vi "DPOAE-CPMR-3.vi"() -> ()   [LabVIEW 2014]
uses:
  <vilib>/measure/NI_MABase.lvlib
  <vilib>/DAQmx/configure/trigger.llb/DAQmx Start Trigger (Digital Edge).vi
  <vilib>/DAQmx/configure/timing.llb/DAQmx Timing (Sample Clock).vi
  <vilib>/DAQmx/create/channels.llb/DAQmx Create Channel (AO-Voltage-Basic).vi
  <vilib>/DAQmx/read.llb/DAQmx Read (Analog Wfm 1Chan NSamp).vi
  <resource>/objmgr/daqmx.rc
  <vilib>/DAQmx/write.llb/DAQmx Write (Analog 1D Wfm NChan NSamp).vi
  <vilib>/DAQmx/create/channels.llb/DAQmx Create Channel (AI-Sound Pressure-Microphone).vi
panel:
  out "Test settings str":string[][](array[string])
  out "Expinfo words":string[](array[string])
  in  "Stop!":bool
  out "End of test":bool
  out "Theoretical freq DPOAE (kHz)":dbl
  out "Frequency Spectrum":cluster{"x0":dbl, "dx":dbl, "magnitude":dbl[]}(graph) caption="spectrum"
  in  "Frequency 2 (kHz)":dbl(ring)=2000.0 items=["0"=0.0, "2"=2000.0, "3"=3000.0, "4"=4000.0, "5"=5000.0, "6"=6000.0, "7"=7000.0, "8"=8000.0, "9"=9000.0, "10"=10000.0, "11"=11000.0, "12"=12000.0, "16"=16000.0]
  out "Stimulus 2 Graph":waveform(dbl)(graph)
  in  "Output Channels (Select two):":tag="PXI1Slot6/ao0:1"
  in  "Amplitude 2":u16(ring)=50 items=["50"=50, "55"=55, "60"=60, "65"=65, "70"=70]
  in  "Add Button 2":bool
  out "Amplitude 1":u16
  out "Frequency 1 (kHz)":dbl=13333.333333333334 format="%#.2f"
  out "Date_Time":string
  out "Main file name":string[](array[string])
  out "Fs":string
  out "File path str":string
  in  "Subject ID":string
  out "Expinfo name":string[](array[string])
  out "File name":string[](array[string])
  in  "File path":path
  in  "User name":string
  in  "Start!":bool
  out "Acquisition Graph":waveform(dbl)(graph)
  in  "Input Channel":tag="PXI1Slot6/ai0"
  out "Fs (#S/s)":dbl
  out "Stimulus 1 Graph":waveform(dbl)(graph)
  out "Current test":i32(knob) scale=0.0..10.0
  in  "Sampling info":cluster{"Fs (#S/s)":dbl, "#S":dbl}={"Fs (#S/s)"=96000.0, "#S"=200000.0}
  out "Protocol list":string[](array[string])
  out "Protocol array settings":dbl[][](array[numeric])
  out "iteration":i32
  in  "How many tests?":i32(slide) scale=0.0..10.0
  out "Protocol words":string[](array[string])
  out "Test settings":dbl[](array[numeric])
  # "Protocol list:"
  # "User, Subject and File settings:"
  # "1"
  # "(without spaces)"
  # "(without spaces)"
  # "(without spaces)"
  # "2"
  # "Choose channels:"
  # "3"
  # "Select sample rate:"
  # "Protocol settings:"
  # "4"
  # "5"
  # "Add a final F2 = 0 kHz stimulus to record noise level."
  # "6"
  # "7"
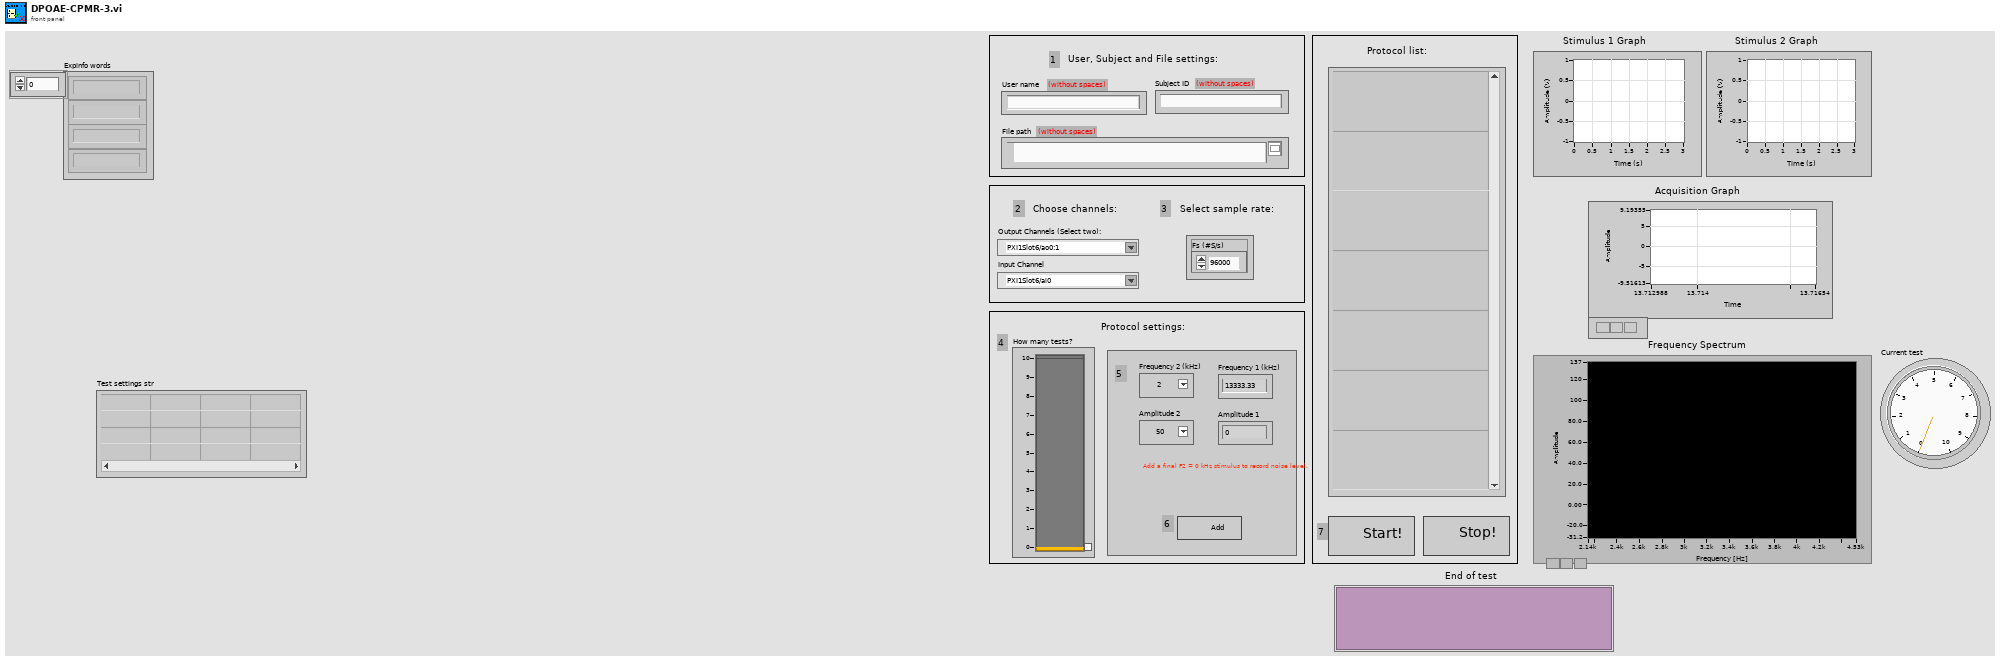
[diagram p1: front panel]
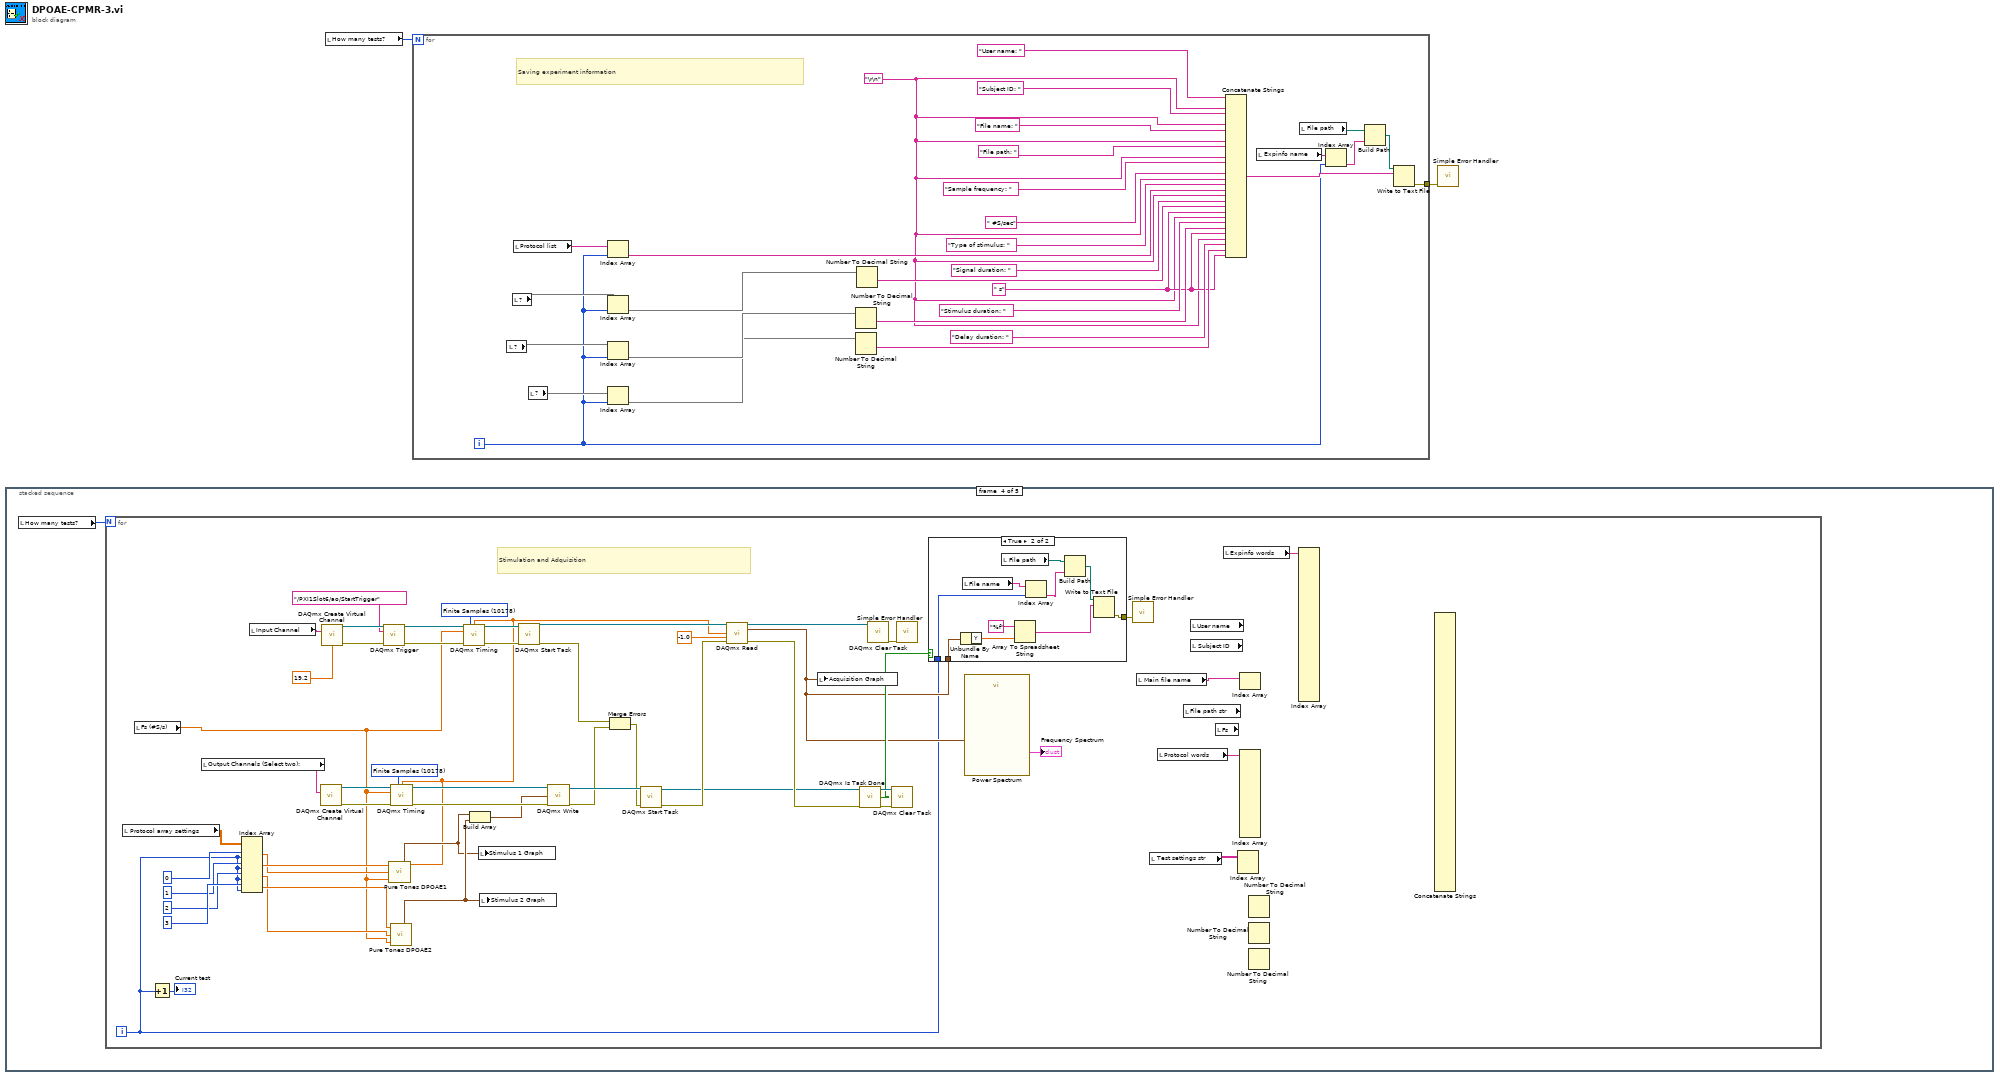
[diagram p0: block diagram]
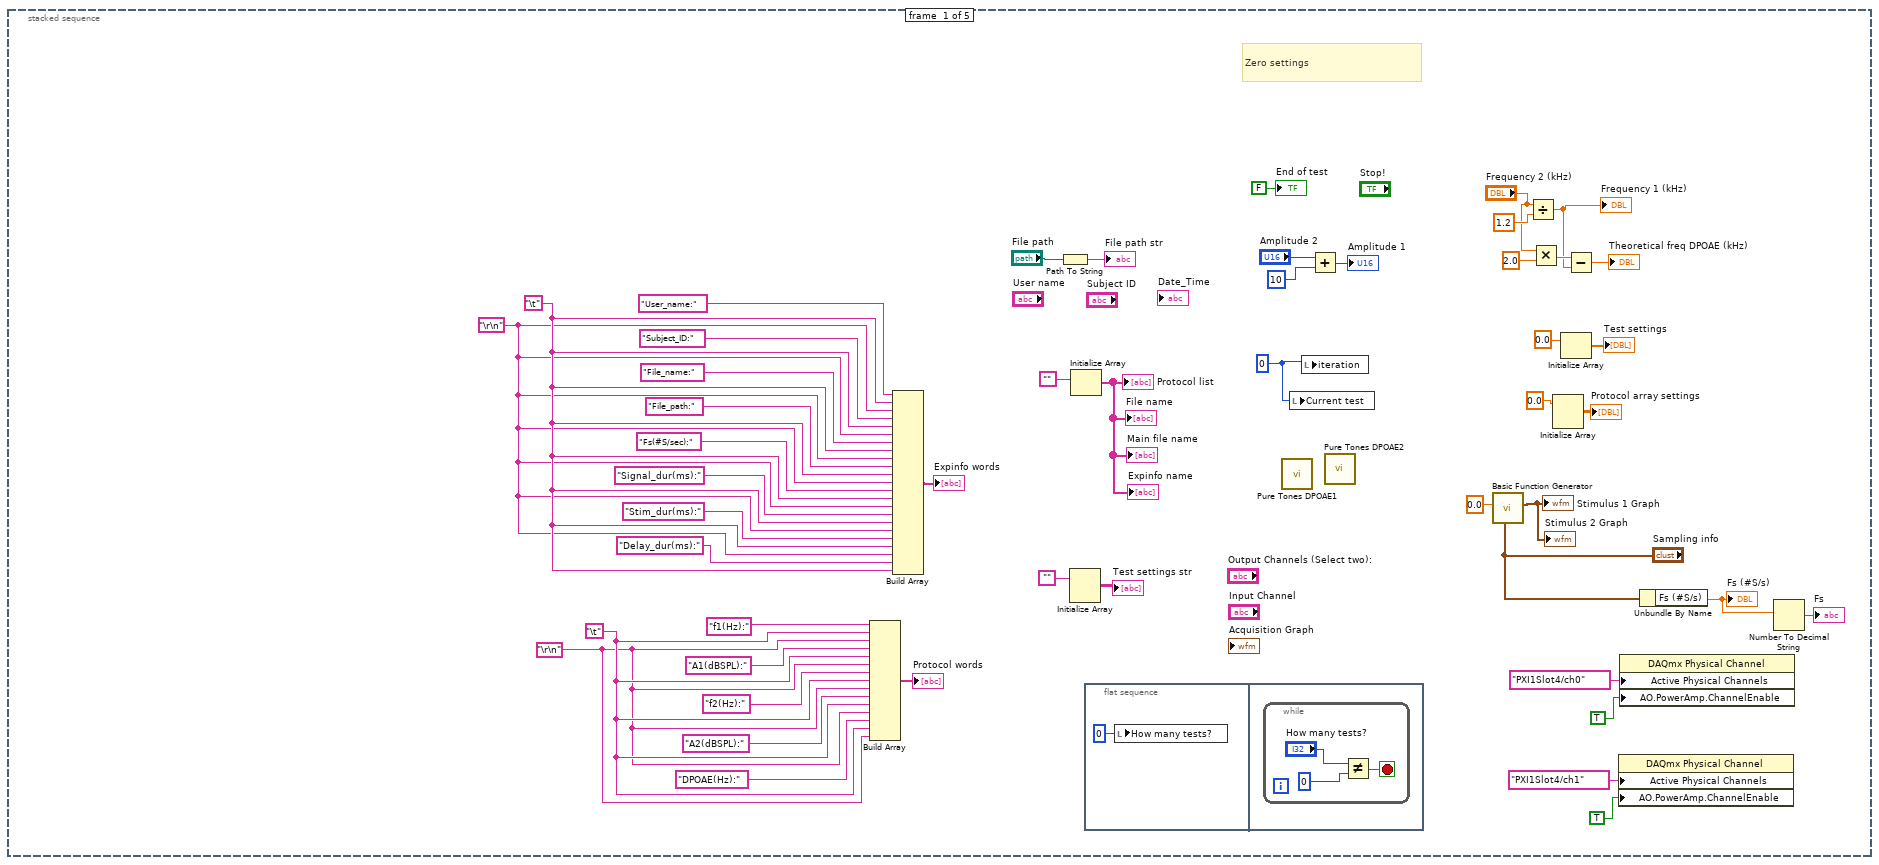
[diagram p2: hidden frame]
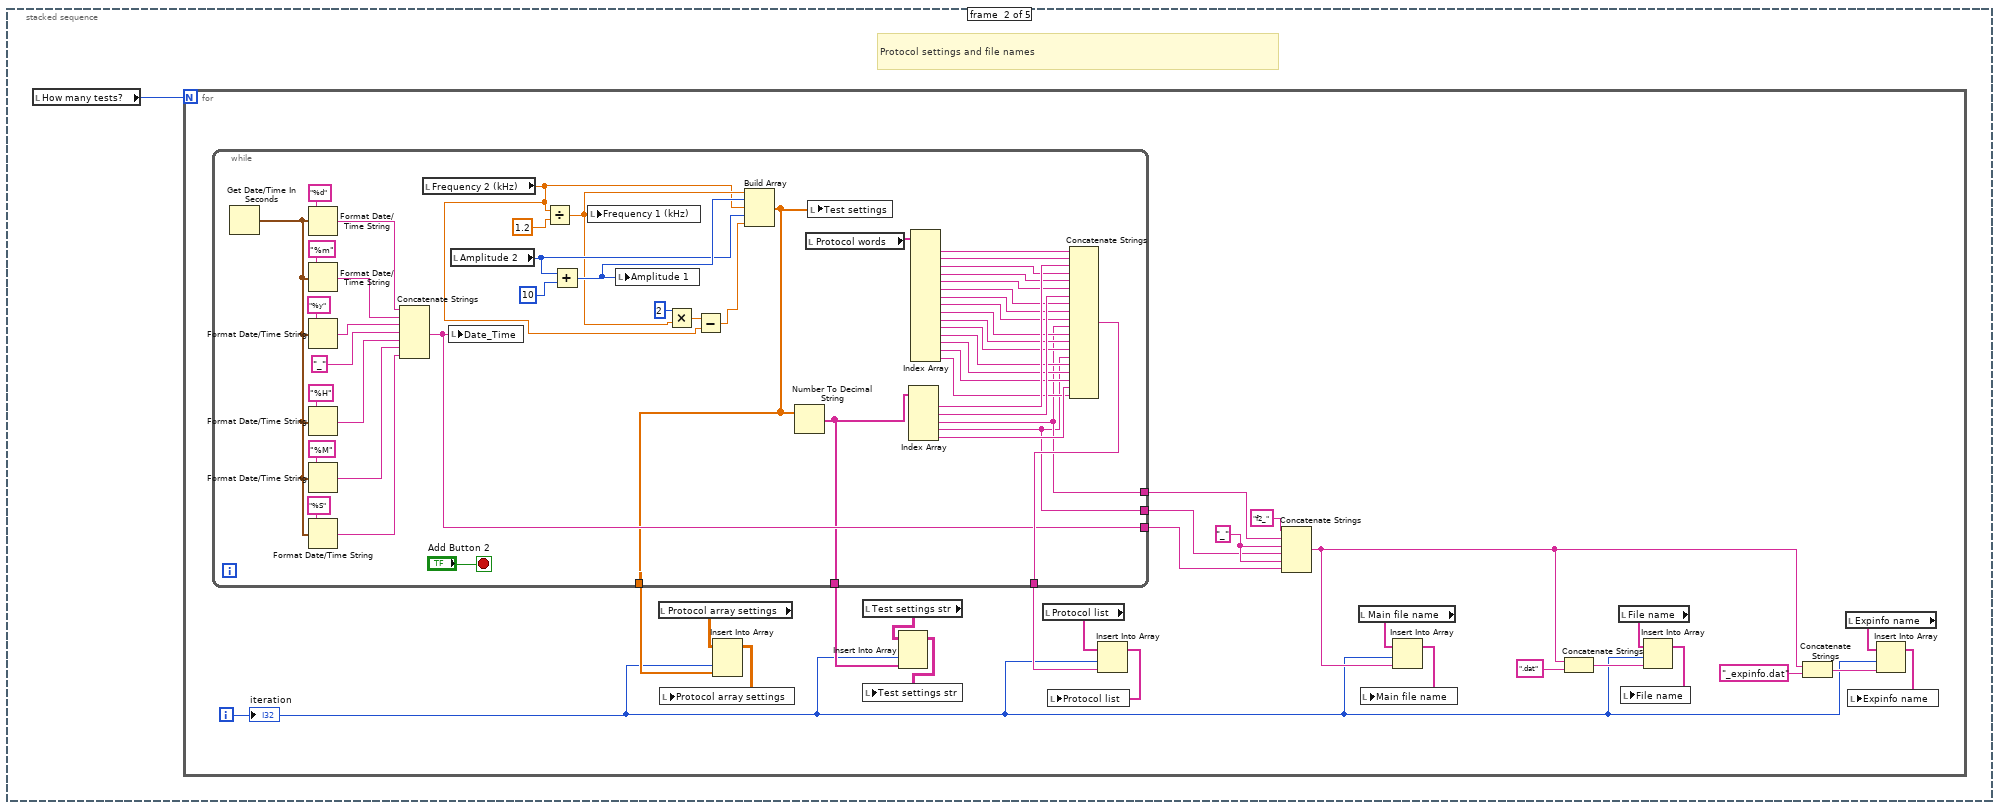
[diagram p3: hidden frame]
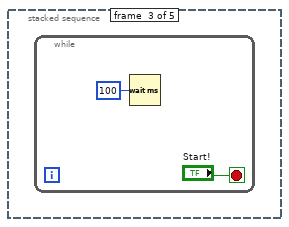
[diagram p4: hidden frame]
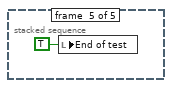
[diagram p6: hidden frame]
diagram:
  n1 = stacked-sequence {
    frame #0 {
      w7 = "\t"
      w6 = "\r\n"
      w11 = "\t"
      w10 = "\r\n"
      w45 = 0 ("iteration")
      # "Zero settings"
      n2 = Build Array("f1(Hz):" ("string"), w7, w6, "A1(dBSPL):", w7, w6, "f2(Hz):" ("string"), w7, w6, "A2(dBSPL):" ("string"), w7, w6, "DPOAE(Hz):" ("string"), w7, w6) -> (→"Protocol words":string[])
      n3 = Build Array("User_name:", w11, w10, "Subject_ID:", w11, w10, "File_name:", w11, w10, "File_path:", w11, w10, "Fs(#S/sec):", w11, w10, "Signal_dur(ms):", w11, w10, "Stim_dur(ms):", w11, w10, "Delay_dur(ms):", w11) -> (→"Expinfo words":string[])
      n4 = Path To String(path="File path") -> (string=→"File path str":string)
      n5 = Initialize Array("") -> (→"Test settings str":string[][])  [unwired: 2 in]
      n6 = Initialize Array("") -> (→"Protocol list" →"File name" →"Expinfo name" →"Main file name":string[])  [unwired: 1 in]
      n7 = flat-sequence {
        frame #0 {
          n8 = local write "How many tests?"(0 ("How many tests?")) -> ()
        }
        frame #1 {
          n9 = while {
            stop <- w54 stop-if-true
            n10 = Not Equal?(x="How many tests?", y=0) -> (x != y?=w54:bool)
          }
        }
      }
      n11 = call <userlib>:"Pure Tones DPOAE1.vi"() -> ()  [unwired: 3 in, 5 out]
      n12 = local write "Current test"(w45) -> ()
      n13 = local write "iteration"(w45) -> ()
      n14 = Add(x="Amplitude 2", y=10) -> (x+y=→"Amplitude 1":i32)
      n15 = call <userlib>:"Pure Tones DPOAE2.vi"() -> ()  [unwired: 3 in, 5 out]
      n16 = call <vilib>:"Basic Function Generator.vi"("sampling info"="Sampling info", "amplitude"=0.0) -> ("signal out"=→"Stimulus 1 Graph" →"Stimulus 2 Graph":waveform(dbl))  [unwired: 7 in, 2 out]
      n17 = Divide(x="Frequency 2 (kHz)", y=1.2) -> (x/y=w26:dbl)
      "Frequency 1 (kHz)" <- w26
      n18 = Multiply(x="Frequency 2 (kHz)", y=2.0) -> (x*y=w27:dbl)
      n19 = Initialize Array(0.0 ("element")) -> (→"Protocol array settings":dbl[][])  [unwired: 2 in]
      n20 = Initialize Array(0.0 ("element")) -> (→"Test settings":dbl[])  [unwired: 1 in]
      n21 = Subtract(x=w27, y=w26) -> (x-y=→"Theoretical freq DPOAE (kHz)":dbl)
      n22 = property class="DAQmx Physical Channel"("Active Physical Channels"=tag "PXI1Slot4/ch1" ("ActivePhysicalChans"), "AO.PowerAmp.ChannelEnable"=TRUE) -> ()  [unwired: 2 in, 2 out]
      n23 = property class="DAQmx Physical Channel"("Active Physical Channels"=tag "PXI1Slot4/ch0" ("ActivePhysicalChans"), "AO.PowerAmp.ChannelEnable"=TRUE) -> ()  [unwired: 2 in, 2 out]
      n24 = Unbundle By Name("Sampling info") -> ("Fs (#S/s)"=w41:dbl)
      "Fs (#S/s)" <- w41
      n25 = Number To Decimal String(number=w41) -> (decimal integer string=→"Fs":string)  [unwired: 1 in]
      "End of test" <- FALSE ("End of test")
    }
    frame #1 {
      # "Protocol settings and file names"
      n26 = local read "How many tests?"() -> (w56:i32)
      n27 = for {
        N: w56 -> [_]
        i -> [w58]
        w72 = "_"
        n28 = while {
          tunnel: [w131] -> w73
          tunnel: [w112] -> w78
          tunnel: [w83] -> w70
          tunnel: [w84] -> w71
          tunnel: [w116] -> w69
          tunnel: [w85] -> w59
          stop <- "Add Button 2" stop-if-true
          n29 = Get Date/Time In Seconds() -> (seconds since 1Jan1904=w123:timestamp)
          n30 = Format Date/Time String(time format string (%c)="%d", seconds (now)=w123) -> (date/time string=w124:string)  [unwired: 1 in]
          n31 = Format Date/Time String(time format string (%c)="%m", seconds (now)=w123) -> (date/time string=w125:string)  [unwired: 1 in]
          n32 = Format Date/Time String(time format string (%c)="%y", seconds (now)=w123) -> (date/time string=w126:string)  [unwired: 1 in]
          n33 = Format Date/Time String(time format string (%c)="%H", seconds (now)=w123) -> (date/time string=w127:string)  [unwired: 1 in]
          n34 = Format Date/Time String(time format string (%c)="%M", seconds (now)=w123) -> (date/time string=w128:string)  [unwired: 1 in]
          n35 = Format Date/Time String(time format string (%c)="%S", seconds (now)=w123) -> (date/time string=w129:string)  [unwired: 1 in]
          n36 = Concatenate Strings(w124, w125, w126, "_", w127, w128, w129) -> (w116:string)
          n37 = local read "Frequency 2 (kHz)"() -> (w106:dbl)
          n38 = local write "Date_Time"(w116) -> ()
          n39 = local read "Amplitude 2"() -> (w113:u16)
          n40 = Divide(x=w106, y=1.2) -> (x/y=w108:dbl)
          n41 = Add(x=w113, y=10) -> (x+y=w114:i32)
          n42 = local write "Frequency 1 (kHz)"(w108) -> ()
          n43 = local write "Amplitude 1"(w114) -> ()
          n44 = Multiply(x=2, y=w108) -> (x*y=w107:dbl)
          n45 = Subtract(x=w107, y=w106) -> (x-y=w105:dbl)
          n46 = Build Array(w108, w114, w106, w113, w105) -> (w112:dbl[])
          n47 = Number To Decimal String(number=w112) -> (decimal integer string=w85:string[])  [unwired: 1 in]
          n48 = local read "Protocol words"() -> (w104:string[])
          n49 = local write "Test settings"(w112) -> ()
          n50 = Index Array(array=w85) -> (element #1=w101:string, element #2=w97:string, element #3=w84:string, element #4=w83:string, element #5=w87:string)  [unwired: 5 in]
          n51 = Index Array(array=w104) -> (element #1=w103:string, element #2=w102:string, element #3=w100:string, element #4=w99:string, element #5=w98:string, element #6=w96:string, element #7=w95:string, element #8=w94:string, element #9=w93:string, element #10=w92:string, element #11=w91:string, element #12=w90:string, element #13=w89:string, element #14=w88:string, element #15=w86:string)  [unwired: 15 in]
          n52 = Concatenate Strings(w103, w102, w101, w100, w99, w98, w97, w96, w95, w94, w84, w93, w92, w91, w83, w90, w89, w88, w87, w86) -> (w131:string)
        }
        n53 = local read "Protocol array settings"() -> (w82:dbl[][])
        n54 = Insert Into Array(array=w82, index (col)=w58, new element=w78) -> (w81:dbl[][])  [unwired: 1 in]
        n55 = local write "Protocol array settings"(w81) -> ()
        n56 = local read "Test settings str"() -> (w60:string[][])
        n57 = Insert Into Array(array=w60, index (col)=w58, new element=w59) -> (w61:string[][])  [unwired: 1 in]
        n58 = local write "Test settings str"(w61) -> ()
        n59 = local read "Protocol list"() -> (w80:string[])
        n60 = Insert Into Array(array=w80, index=w58, new element=w73) -> (w79:string[])
        n61 = local write "Protocol list"(w79) -> ()
        n62 = Concatenate Strings("f2_" ("string"), w71, w72, w70, w72, w69) -> (w66:string)
        n63 = local read "Main file name"() -> (w68:string[])
        n64 = Insert Into Array(array=w68, index=w58, new element=w66) -> (w67:string[])
        n65 = local write "Main file name"(w67) -> ()
        n66 = Concatenate Strings(w66, ".dat") -> (w62:string)
        n67 = local read "File name"() -> (w65:string[])
        n68 = Insert Into Array(array=w65, index=w58, new element=w62) -> (w64:string[])
        n69 = local write "File name"(w64) -> ()
        n70 = Concatenate Strings(w66, "_expinfo.dat") -> (w74:string)
        n71 = local read "Expinfo name"() -> (w76:string[])
        n72 = Insert Into Array(array=w76, index=w58, new element=w74) -> (w77:string[])
        n73 = local write "Expinfo name"(w77) -> ()
        "iteration" <- w58
      }
    }
    frame #2 {
      n74 = while {
        stop <- "Start!" stop-if-true
        n75 = Wait (ms)(milliseconds to wait=u32 100) -> ()  [unwired: 1 out]
      }
    }
    frame #3 {
      n76 = local read "How many tests?"() -> (w134:i32)
      n77 = for {
        N: w134 -> [_]
        i -> [w139]
        w173 = 10178 items=["Finite Samples"=10178, "Continuous Samples"=10123, "Hardware Timed Single Point"=12522] ("sample mode")
        w178 = 10178 items=["Finite Samples"=10178, "Continuous Samples"=10123, "Hardware Timed Single Point"=12522] ("sample mode")
        # "Stimulation and Adquisition"
        n78 = local read "Protocol array settings"() -> (w183:dbl[][])
        n79 = local read "Fs (#S/s)"() -> (w143:dbl)
        n80 = Increment(x=w139) -> (x+1=→"Current test":i32)
        n81 = local read "Output Channels (Select two):"() -> (w165:tag)
        n82 = Index Array(array=w183, index (row) #1=0 ("disabled index (row)"), index (col) #1=w139, index (row) #2=1, index (col) #2=w139, index (row) #3=2, index (col) #3=w139, index (row) #4=3, index (col) #4=w139) -> (element #1=w144:dbl, element #2=w145:dbl, element #3=w149:dbl, element #4=w150:dbl)
        n83 = local read "Input Channel"() -> (w182:tag)
        n84 = call-poly <vilib>:"DAQmx Create Virtual Channel.vi"("physical channels"=w165) -> ("task out"=w167:refnum<k21>, "error out"=w166:errorcluster)  [unwired: 13 in]
        n85 = call-poly <vilib>:"DAQmx Create Virtual Channel.vi"("physical channels"=w182, "microphone sensitivity"=19.2) -> ("task out"=w180:refnum<k21>, "error out"=w181:errorcluster)  [unwired: 12 in]
        n86 = call-poly <vilib>:"DAQmx Trigger.vi"("task/channels in"=w180, "source"=tag "/PXI1Slot6/ao/StartTrigger", "error in"=w181) -> ("task out"=w176:refnum<k21>, "error out"=w177:errorcluster)  [unwired: 11 in]
        n87 = call <userlib>:"Pure Tones DPOAE1.vi"("Amplitude (dB SPL)"=w145, "Frequency (Hz)"=w144, "Fs (#S/s)"=w143) -> ("Signal duration (#S)"=w146:dbl, "Stimulus Waveform"=w147:waveform(dbl))  [unwired: 3 out]
        n88 = call <userlib>:"Pure Tones DPOAE2.vi"("Amplitude (dB SPL)"=w150, "Frequency (Hz)"=w149, "Fs (#S/s)"=w143) -> ("Stimulus Waveform"=w151:waveform(dbl))  [unwired: 4 out]
        n89 = call-poly <vilib>:"DAQmx Timing.vi"("task/channels in"=w167, "sample mode"=w173, "samples per channel"=w146, "rate"=w143, "error in"=w166) -> ("task out"=w171:refnum<k21>, "error out"=w172:errorcluster)  [unwired: 9 in]
        n90 = call-poly <vilib>:"DAQmx Timing.vi"("task/channels in"=w176, "sample mode"=w178, "samples per channel"=w146, "rate"=w143, "error in"=w177) -> ("task out"=w174:refnum<k21>, "error out"=w175:errorcluster)  [unwired: 9 in]
        n91 = Build Array(w147, w151) -> (w153:waveform(dbl)[])
        n92 = local write "Stimulus 1 Graph"(w147) -> ()
        n93 = local write "Stimulus 2 Graph"(w151) -> ()
        n94 = call <vilib>:"DAQmx Start Task.vi"("task/channels in"=w174, "error in"=w175) -> ("task out"=w169:refnum<k21>, "error out"=w163:errorcluster)  [unwired: 12 in]
        n95 = call-poly <vilib>:"DAQmx Write.vi"("task/channels in"=w171, "data"=w153, "error in"=w172) -> ("task out"=w170:refnum<k21>, "error out"=w162:errorcluster)  [unwired: 10 in, 1 out]
        n96 = Merge Errors(w163, w162) -> (w161:errorcluster)
        n97 = call <vilib>:"DAQmx Start Task.vi"("task/channels in"=w170, "error in"=w161) -> ("task out"=w156:refnum<k21>, "error out"=w160:errorcluster)  [unwired: 12 in]
        n98 = call-poly <vilib>:"DAQmx Read.vi"("task/channels in"=w169, "number of samples per channel"=w146, "timeout"=-1.0, "error in"=w160) -> ("task out"=w155:refnum<k21>, "data"=w140:waveform(dbl), "error out"=w159:errorcluster)  [unwired: 9 in]
        n99 = local write "Acquisition Graph"(w140) -> ()
        n100 = call <vilib>:"DAQmx Is Task Done.vi"("task/channels in"=w156, "error in"=w159) -> ("task out"=w157:refnum<k21>, "task done?"=w148:bool, "error out"=w158:errorcluster)  [unwired: 11 in]
        n101 = call <vilib>:"DAQmx Clear Task.vi"("task in"=w155) -> ("error out"=w168:errorcluster)  [unwired: 14 in]
        n102 = call <vilib>:"DAQmx Clear Task.vi"("task in"=w157, "error in"=w158) -> ()  [unwired: 13 in, 1 out]
        n103 = call <vilib>:"Simple Error Handler.vi"("error in (no error)"=w168) -> ()  [unwired: 4 in, 5 out]
        n104 = case shown="True" w148 {
          tunnel: [_ w195] -> w164
          tunnel: w140 -> [_ w189]
          tunnel: w139 -> [_ w188]
          frame False {
          }
          frame True {
            n105 = Unbundle By Name(w189) -> ("Y"=w190:dbl[])
            n106 = local read "File name"() -> (w197:string[])
            n107 = local read "File path"() -> (w191:path)
            n108 = Array To Spreadsheet String(array=w190, 3:"%f" ("text")) -> (spreadsheet string=w193:string)  [unwired: 1 in]
            n109 = Index Array(array=w197, index=w188) -> (element=w192:string)
            n110 = Build Path(base path=w191, name or relative path=w192) -> (appended path=w196:path)
            n111 = Write to Text File(file (use dialog)=w196, text=w193) -> (error out=w195:errorcluster)  [unwired: 2 in, 2 out]
          }
        }
        n112 = call "Power Spectrum"("input signal"=w140) -> ("spectrum"=→"Frequency Spectrum":cluster{"x0":dbl, "dx":dbl, "magnitude":dbl[]})  [unwired: 13 in, 5 out]
        n113 = call <vilib>:"Simple Error Handler.vi"("error in (no error)"=w164) -> ()  [unwired: 4 in, 5 out]
        n114 = local read "Main file name"() -> (w137:string[])
        n115 = local read "Test settings str"() -> (w135:string[][])
        n116 = local read "Protocol words"() -> (w136:string[])
        n117 = local read "File path str"() -> ()  [unwired: 1 out]
        n118 = local read "User name"() -> ()  [unwired: 1 out]
        n119 = local read "Subject ID"() -> ()  [unwired: 1 out]
        n120 = local read "Fs"() -> ()  [unwired: 1 out]
        n121 = local read "Expinfo words"() -> (w138:string[])
        n122 = Index Array(array=w135) -> ()  [unwired: 2 in, 1 out]
        n123 = Index Array(array=w137) -> ()  [unwired: 1 in, 1 out]
        n124 = Index Array(array=w136) -> ()  [unwired: 14 in, 14 out]
        n125 = Number To Decimal String() -> ()  [unwired: 2 in, 1 out]
        n126 = Number To Decimal String() -> ()  [unwired: 2 in, 1 out]
        n127 = Number To Decimal String() -> ()  [unwired: 2 in, 1 out]
        n128 = Index Array(array=w138) -> ()  [unwired: 26 in, 26 out]
        n129 = Concatenate Strings() -> ()  [unwired: 51 in, 1 out]
      }
    }
    frame #4 {
      n130 = local write "End of test"(TRUE) -> ()
    }
  }
  n131 = local read "How many tests?"() -> (w2:i32)
  n132 = for {
    N: w2 -> [_]
    tunnel: [w210] -> w1
    i -> [w201]
    w214 = " s"
    w199 = "\r\n"
    # "Saving experiment information"
    n133 = local read item#-1() -> (w204)
    n134 = local read item#-1() -> (w206)
    n135 = local read "Protocol list"() -> (w222:string[])
    n136 = local read item#-1() -> (w202)
    n137 = Index Array(array=w222, index=w201) -> (element=w221:string)
    n138 = Index Array(array=w206, index=w201) -> (element=w205)
    n139 = Index Array(array=w204, index=w201) -> (element=w203)
    n140 = Index Array(array=w202, index=w201) -> (element=w200)
    n141 = Number To Decimal String(number=w203) -> (decimal integer string=w217:string)  [unwired: 1 in]
    n142 = Number To Decimal String(number=w200) -> (decimal integer string=w215:string)  [unwired: 1 in]
    n143 = Number To Decimal String(number=w205) -> (decimal integer string=w219:string)  [unwired: 1 in]
    n144 = Concatenate Strings("User name: ", w199, "Subject ID: ", w199, "File name: ", w199, "File path: ", w199, "Sample frequency: ", " #S/sec", w199, "Type of stimulus: ", w221, w199, "Signal duration: ", w219, w214, w199, "Stimulus duration: ", w217, w214, w199, "Delay duration: ", w215, w214) -> (w209:string, w229:string, w228:string, w227:string, w208:string, w225:string)
    n145 = local read "Expinfo name"() -> (w211:string[])
    n146 = local read "File path"() -> (w207:path)
    n147 = Index Array(array=w211, index=w201) -> (element=w213:string)
    n148 = Build Path(base path=w207, name or relative path=w213) -> (appended path=w212:path)
    n149 = Write to Text File(file (use dialog)=w212, text=w209) -> (error out=w210:errorcluster)  [unwired: 2 in, 2 out]
  }
  n150 = call <vilib>:"Simple Error Handler.vi"("error in (no error)"=w1) -> ()  [unwired: 4 in, 5 out]
